vi "Clutster to list transfer.vi"() -> ()   [LabVIEW 2012]
uses:
  Volvo/Controls/Volvo States.ctl
  Volvo/Controls/Volvo Tests.ctl
panel:
  out "Array 3":string[][](array[string])
  out "Array 2":T1[](array[typedef])
  in  "Message":T1
  out "element":string
  in  "stop":bool
  in  "Listbox":i32(listbox)
  out "Array":string[](array[string])
  in  "Testplan":T2={"Communications"=TRUE, "Fault Report"=TRUE, "Initialize"=FALSE, "PTC Power Ctrl"=FALSE, "PTC Rod Trigger"=FALSE, "PTC Rod Ripple"=FALSE, "Active Low PTC Ctrl"=FALSE, "Max Ramp Rate"=FALSE, "Warm Restart"=TRUE, "Error Count"=TRUE, "Critical Fault Protect"=FALSE, "Critical Fault Report"=FALSE, "Open Load"=FALSE, "Short Circuits"=FALSE, "High Ohmic"=FALSE, "PCB over Temp"=FALSE, "Instant Switch Off"=FALSE, "Voltage OOS"=FALSE}
  out "TestPlan":i32(listbox)
  in  "Add Test":bool
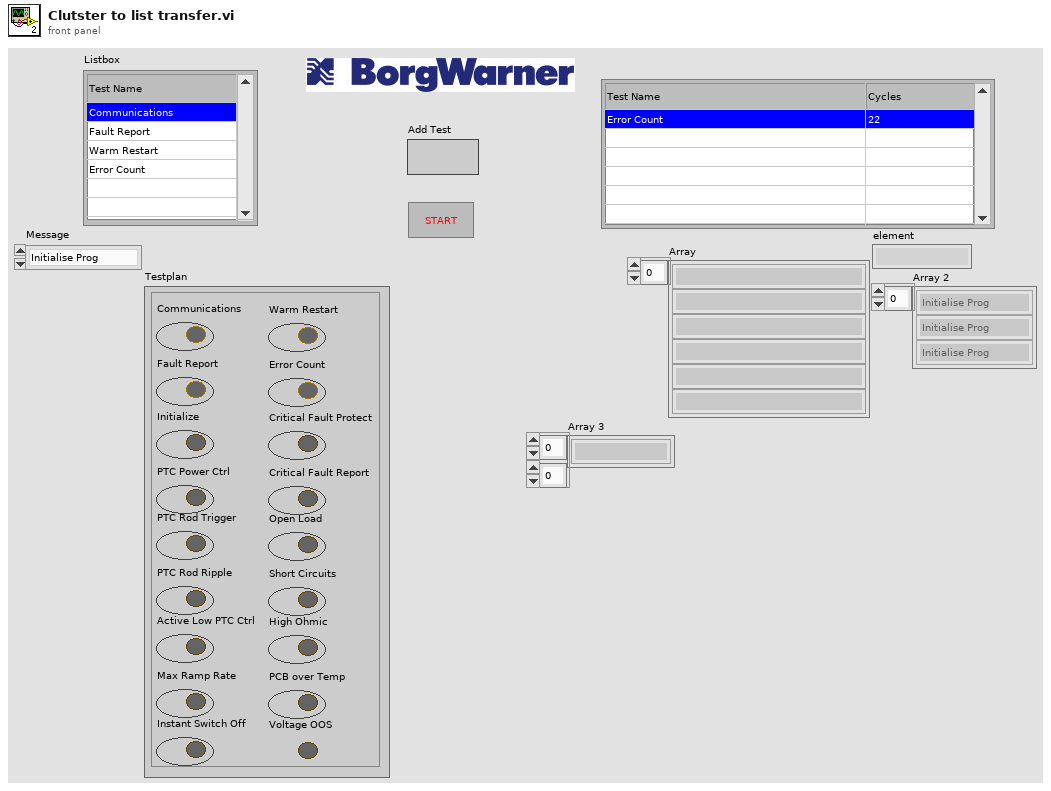
[diagram p1: front panel]
types:
  T1 = typedef "Volvo States.ctl" = enum16{"Initialise Prog", "Exit", "UpdateDisplay", "Error", "UpdateTestplan", "Confirm Quit", "Communications", "Fault Report", "Initialize", "PTC Power Ctrl", "PTC Rod Trigger", "Active Low PTC Ctrl", "Max Ramp Rate", "Immediate Switch Off", "Warm Restart", "Error Count", "Critical Fault Protect", "Critical Fault Report", "Open Load", "Short Circuits", "High Ohmic", "PCB over Temp", "Voltage OOS"}
  T2 = typedef "Volvo Tests.ctl" = cluster{"Communications":bool, "Fault Report":bool, "Initialize":bool, "PTC Power Ctrl":bool, "PTC Rod Trigger":bool, "PTC Rod Ripple":bool, "Active Low PTC Ctrl":bool, "Max Ramp Rate":bool, "Warm Restart":bool, "Error Count":bool, "Critical Fault Protect":bool, "Critical Fault Report":bool, "Open Load":bool, "Short Circuits":bool, "High Ohmic":bool, "PCB over Temp":bool, "Instant Switch Off":bool, "Voltage OOS":bool}
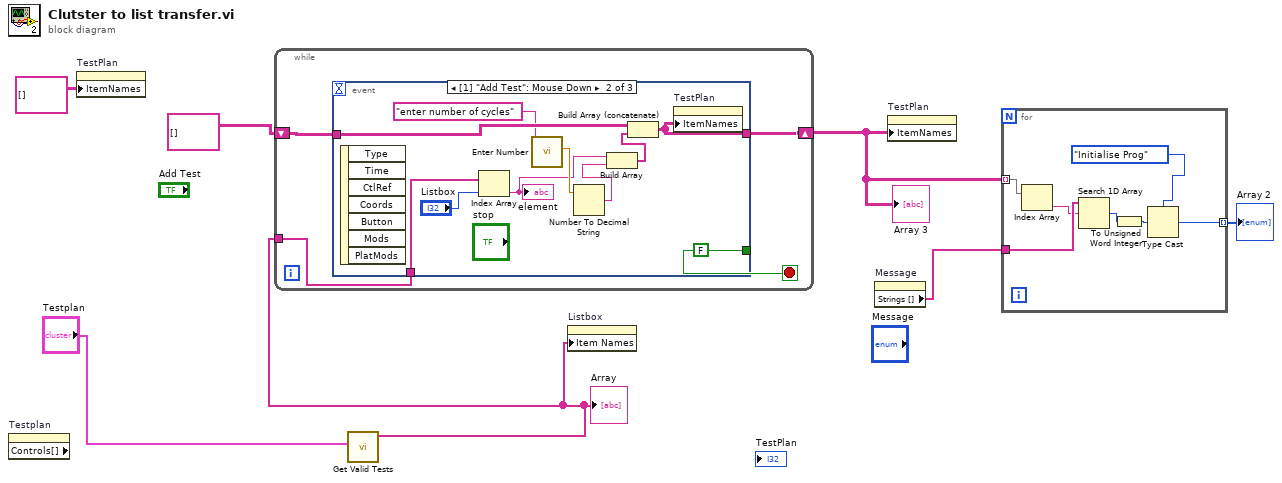
[diagram p0: block diagram]
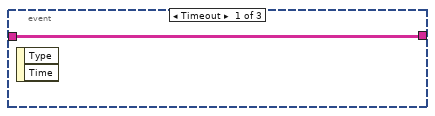
[diagram p2: hidden frame]
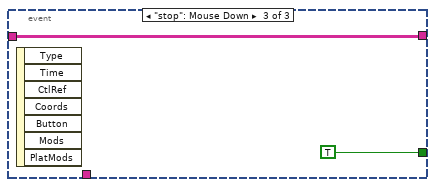
[diagram p3: hidden frame]
diagram:
  n1 = property on="Testplan" class="Clust (strict)"() -> ("Controls[]"=w8:refnum<vi>[])  [unwired: 2 in, 2 out]
  n2 = property on="TestPlan" class="MCListbox (strict)"("ItemNames"=string[][] [] ("Item Names")) -> ()  [unwired: 2 in, 2 out]
  n3 = call "Get Valid Tests.vi"("Testplan"="Testplan") -> ("Array"=w7:string[])  [unwired: 9 in, 1 out]
  "Array" <- w7
  n4 = while {
    tunnel: w7 -> [w11]
    shift-right: [w10] -> w3
    shift-left: string[][] [] -> [w9]
    stop <- w12 stop-if-true
    n5 = event shown="[1] \"Add Test\": Mouse Down" {
      selector: _ -> [_ _ _]
      dyn-events: _ -> [_ _ _]
      timeout: _ -> [_ _ _]
      tunnel: [_ FALSE ("stop") TRUE ("stop")] -> w12
      tunnel: w11 -> [_ w21 _]
      tunnel: [w13 w14 w24] -> w10
      tunnel: w9 -> [w13 w22 w24]
      event Timeout {
        n6 = event-data() -> ()  [unwired: 1 in, 2 out]
      }
      event "Add Test": Mouse Down {
        n7 = event-data() -> ()  [unwired: 1 in, 7 out]
        n8 = Index Array(array=w21, index="Listbox") -> (element=w18:string)
        "element" <- w18
        n9 = call "Enter Number.vi"("Message"="enter number of cycles") -> ("Numeric Value"=w19:dbl)  [unwired: 9 in, 1 out]
        n10 = Number To Decimal String(number=w19) -> (decimal integer string=w17:string)  [unwired: 1 in]
        n11 = Build Array(w18, w17) -> (w16:string[])
        n12 = Build Array (concatenate)(w22, w16) -> (w14:string[][])
        n13 = property on="TestPlan" class="MCListbox (strict)"("ItemNames"=w14) -> ()  [unwired: 2 in, 2 out]
      }
      event "stop": Mouse Down {
        n14 = event-data() -> ()  [unwired: 1 in, 7 out]
      }
    }
  }
  "Array 3" <- w3
  n15 = property on="Listbox" class="LstBox (strict)"("Item Names"=w7) -> ()  [unwired: 2 in, 2 out]
  n16 = property on="Message" class="Enum (strict)"() -> ("Strings []"=w4:string[])  [unwired: 2 in, 2 out]
  n17 = property on="TestPlan" class="MCListbox (strict)"("ItemNames"=w3) -> ()  [unwired: 2 in, 2 out]
  n18 = for {
    tunnel: w4 -> [w32]
    tunnel: w3 -> [w31] mode=indexing
    tunnel: [w29] -> w2 mode=indexing
    n19 = Index Array(array=w31) -> (element=w30:string)  [unwired: 1 in]
    n20 = Search 1D Array(1D array=w32, element=w30) -> (index of element=w27:i32)  [unwired: 1 in]
    n21 = To Unsigned Word Integer(number=w27) -> (unsigned 16bit integer=w26:u16)
    n22 = Type Cast(type=Volvo_States."Initialise Prog" ("Message"), x=w26) -> (*(type *) &x=w29:T1)
  }
  "Array 2" <- w2
